vi "fpga_Calculate Timestamp.vi"(0 "resample data and position":T1 {"frequency" format="%.59g"; "Resample position" format="%.53g"; "even-angle signal" format="%.30g"}, 1 "timestamp&count":T3 {"TAI timestamp" format="%.42g"}, 7 "muti_ch position valid?":bool, 9 "input valid":bool, 12 "ready for output":bool) -> (4 "Resample data and time":T2, 10 "output valid":bool, 14 "ready for input":bool)   [LabVIEW 2011, in "NI_EP_Resample_FPGA.lvlib"]
uses:
  <vilib>/addons/Electrical Power/PQ/Resampling/NI_EP_Resample_FPGA.lvlib
  <vilib>/addons/Electrical Power/PQ/Resampling/FPGA/subVIs/fpga_Resampled.ctl
  <vilib>/rvi/FXPMathLib/FxpSub/subVIs/nifxpmath_Sub_SimConfig.ctl
  <vilib>/fxp/LVFixedPointQuantizationPolicyTypeDef.ctl
  <vilib>/fxp/LVFixedPointOverflowPolicyTypeDef.ctl
  <vilib>/rvi/FXPMathLib/FxpSub/simVIs/DllFxpSubTemp_sub.vi
  <vilib>/rvi/FXPMathLib/FxpSub/XNode/nifxpmath_Sub.xnode
  <vilib>/rvi/FXPMathLib/FxpMul/XNode/nifxpmath_Multiplier.xnode
  <vilib>/rvi/FXPMathLib/basic elements/FxpDiscreteDelay/XNode/nifxpmath_DiscreteDelay.xnode
  <vilib>/rvi/FXPMathLib/sim/FxpSim.dll
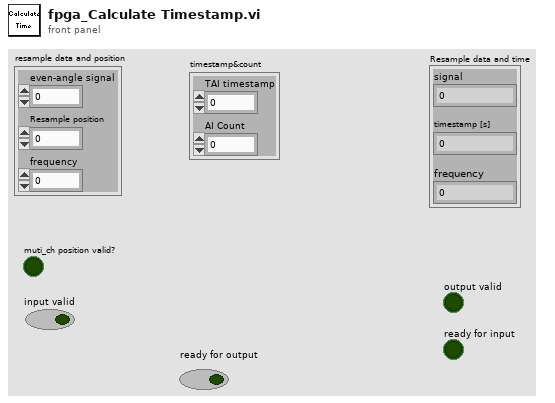
[diagram p1: front panel]
types:
  T1 = cluster{"even-angle signal":fxp<+/-,32,3>, "Resample position":fxp<+,64,16>, "frequency":fxp<+,32,8>}
  T2 = typedef "NI_EP_Resample_FPGA.lvlib/fpga_Resampled.ctl" = cluster{"signal":fxp<+/-,32,3>, "timestamp [s]":fxp<+,64,32>, "frequency":fxp<+,32,8>}
  T3 = cluster{"TAI timestamp":fxp<+,64,32>, "AI Count":u16}
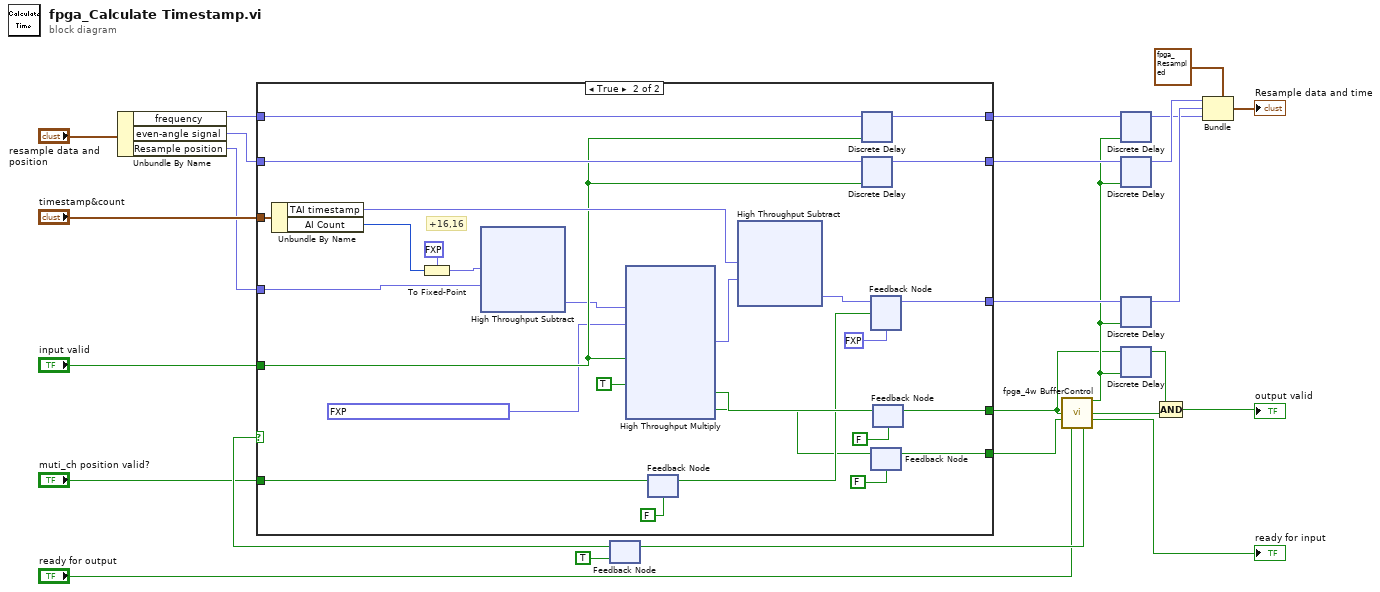
[diagram p0: block diagram]
diagram:
  n1 = Unbundle By Name("resample data and position") -> ("frequency"=w4:fxp<+,32,8>, "even-angle signal"=w3:fxp<+/-,32,3>, "Resample position"=w2:fxp<+,64,16>)
  n2 = feedback #1(TRUE ("logic enable")) -> (w24:bool)
  n3 = case shown="True" w24 {
    tunnel: "timestamp&count" -> [_ w41]
    tunnel: w3 -> [_ w31]
    tunnel: w2 -> [_ w40]
    tunnel: w4 -> [_ w33]
    tunnel: "input valid" -> [_ w29]
    tunnel: "muti_ch position valid?" -> [_ w39]
    tunnel: [_ w38] -> w10
    tunnel: [_ w35] -> w15
    tunnel: [_ w32] -> w14
    tunnel: [_ w30] -> w13
    tunnel: [_ w34] -> w12
    frame False {
    }
    frame True {
      # "+16,16"
      n4 = Unbundle By Name(w41) -> ("TAI timestamp"=w51:fxp<+,64,32>, "AI Count"=w42:u16)
      n5 = To Fixed-Point(fixed-point type=fxp<+,16,16> 0.0, number=w42) -> (fixed-point=w52:fxp<+,16,16>)
      n6 = xnode "High Throughput Subtract"("x"=w52, "y"=w40) -> ("x-y"=w27:fxp<+,32,16>)
      n7 = xnode "High Throughput Multiply"("x"=w27, "y"=fxp<+,16,-15> 2.00001522898674e-05 ("Numeric"), "input valid"=w29, "ready for output (T)"=TRUE) -> ("x*y"=w49:fxp<+,64,32>, "output valid"=w46:bool, "ready for input"=w36:bool)
      n8 = feedback #2(FALSE ("muti_ch position valid?")) -> (w45:bool)
      n9 = feedback-in #2(w39) -> ()
      n10 = xnode "High Throughput Subtract"("x"=w51, "y"=w49) -> ("x-y"=w48:fxp<+,64,32>)
      n11 = xnode "Discrete Delay"("D"=w33, "enable"=w29) -> ("Q"=w32:fxp<+,32,8>)
      n12 = xnode "Discrete Delay"("D"=w31, "enable"=w29) -> ("Q"=w30:fxp<+/-,32,3>)
      n13 = feedback #3(fxp<+,64,32> 0.0 ("x-y")) -> (w34:fxp<+,64,32>)
      n14 = feedback-in #3(w48, w45) -> ()
      n15 = feedback #4(FALSE ("output valid")) -> (w35:bool)
      n16 = feedback-in #4(w36) -> ()
      n17 = feedback #5(FALSE ("output valid")) -> (w38:bool)
      n18 = feedback-in #5(w46) -> ()
    }
  }
  n19 = call <vilib>:"fpga_4w BufferControl.vi"("DR"=w10, "RFI"=w15, "RFO"="ready for output") -> ("buff enable"=w11:bool, "output valid"=w21:bool, "ready for input"=→"ready for input":bool, "logic enable"=w26:bool)  [unwired: 9 in]
  n20 = feedback-in #1(w26) -> ()
  n21 = xnode "Discrete Delay"("D"=w14, "enable"=w11) -> ("Q"=w7:fxp<+,32,8>)
  n22 = xnode "Discrete Delay"("D"=w13, "enable"=w11) -> ("Q"=w9:fxp<+/-,32,3>)
  n23 = xnode "Discrete Delay"("D"=w12, "enable"=w11) -> ("Q"=w8:fxp<+,64,32>)
  n24 = xnode "Discrete Delay"("D"=w10, "enable"=w11) -> ("Q"=w23:bool)
  n25 = Compound Arithmetic op=AND(w23, w21) -> (→"output valid":bool)
  n26 = Bundle(cluster=T2 {"signal"=0.0, "timestamp [s]"=0.0, "frequency"=0.0} ("Resample data and time"), "signal"=w9, "timestamp [s]"=w8, "frequency"=w7) -> (→"Resample data and time":T2)
